vi "Export2Excel.vi"(8 "进度数值":refnum<vi>, 9 "Slide输入":refnum<vi>, 10 "波形数组":cluster{dbl[], dbl[]}[](array[cluster]), 11 "信号名数组":string[](array[string])) -> ()   [LabVIEW 2015]
uses:
  <vilib>/Utility/NIReport.llb/Append Text Table to Report (wrap).vi
  <vilib>/Utility/NIReport.llb/NI_report.lvclass
panel:
  out "进度数值0":string="0%"
  out "水平进度条":u8(slide) scale=0.0..100.0
  # "正在导出至EXCEL，请稍等"
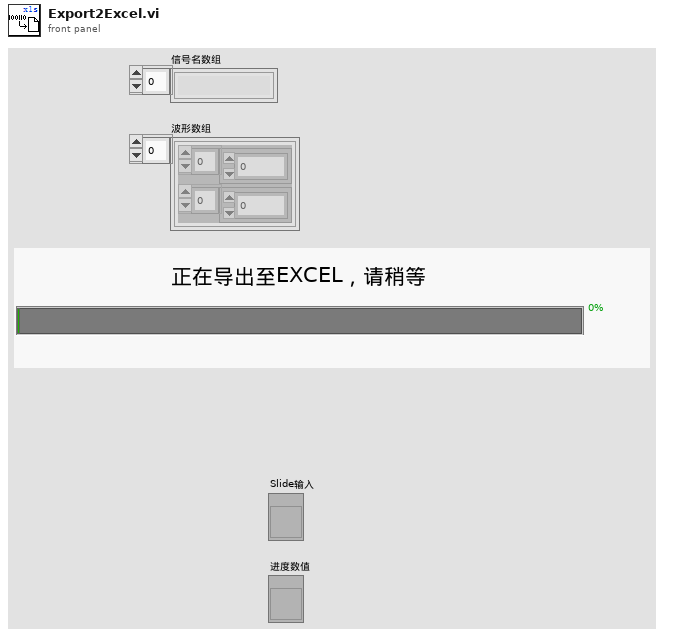
[diagram p1: front panel]
types:
  T1 = enum16{"Standard Report", "HTML", "Word", "Excel"}
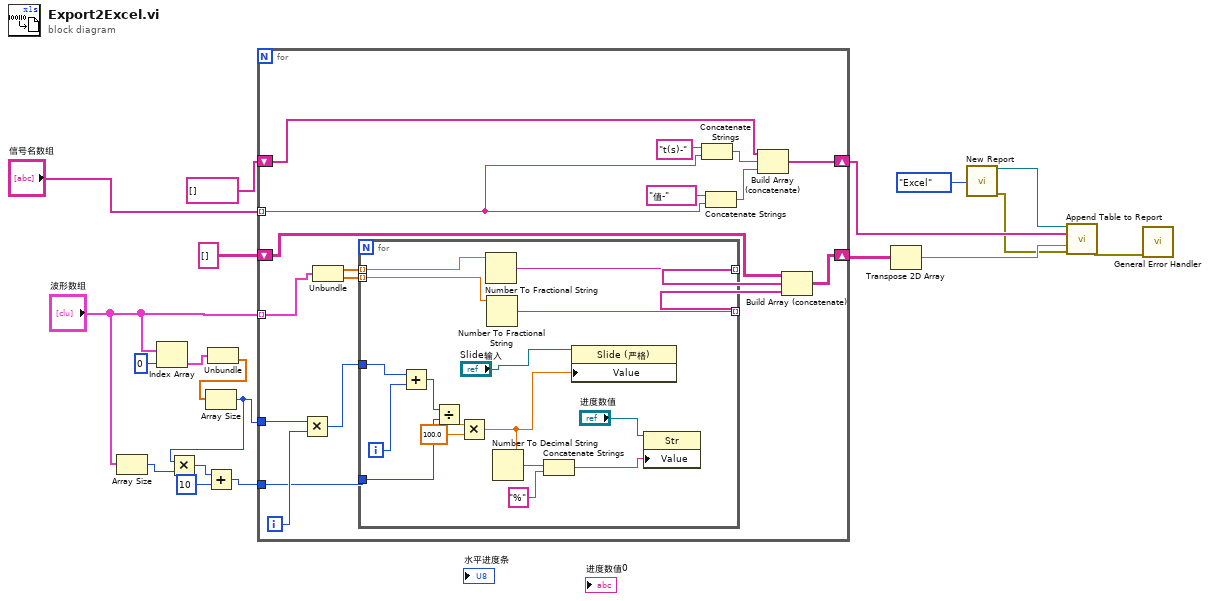
[diagram p0: block diagram]
diagram:
  n1 = Array Size(array="波形数组") -> (size(s)=w7:i32)
  n2 = Index Array(array="波形数组", index=0 ("索引")) -> (element=w9:cluster{dbl[], dbl[]})
  n3 = Unbundle(w9) -> (w8:dbl[])  [unwired: 1 out]
  n4 = Array Size(array=w8) -> (size(s)=w6:i32)
  n5 = Multiply(x=w6, y=w7) -> (x*y=w3:i32)
  n6 = Add(x=w3, y=10) -> (x+y=w2:i32)
  n7 = for {
    tunnel: "波形数组" -> [w33] mode=indexing
    shift-right: [w32] -> w13
    shift-left: string[][] [] -> [w31]
    tunnel: "信号名数组" -> [w27] mode=indexing
    shift-right: [w25] -> w19
    shift-left: string[] [] -> [w24]
    tunnel: w6 -> [w22]
    tunnel: w2 -> [w20]
    i -> [w23]
    n8 = Multiply(x=w22, y=w23) -> (x*y=w21:i32)
    n9 = Unbundle(w33) -> (w37:dbl[], w36:dbl[])
    n10 = for {
      tunnel: w37 -> [w53] mode=indexing
      tunnel: w36 -> [w51] mode=indexing
      tunnel: [w52] -> w35 mode=indexing
      tunnel: [w50] -> w34 mode=indexing
      tunnel: w21 -> [w49]
      tunnel: w20 -> [w46]
      i -> [w48]
      n11 = Add(x=w49, y=w48) -> (x+y=w47:i32)
      n12 = Divide(x=w47, y=w46) -> (x/y=w45:dbl)
      n13 = Multiply(x=w45, y=100.0) -> (x*y=w38:dbl)
      n14 = Number To Fractional String(number=w53) -> (F-format string=w52:string)  [unwired: 3 in]
      n15 = Number To Fractional String(number=w51) -> (F-format string=w50:string)  [unwired: 3 in]
      n16 = Number To Decimal String(number=w38) -> (decimal integer string=w43:string)  [unwired: 1 in]
      n17 = Concatenate Strings(w43, "%" ("字符串")) -> (w40:string)
      n18 = property class="Slide (严格)"(reference="Slide输入", "Value"=w38) -> ()  [unwired: 1 in, 2 out]
      n19 = property class="Str"(reference="进度数值", "Value"=w40) -> ()  [unwired: 1 in, 2 out]
    }
    n20 = Concatenate Strings("t(s)-" ("字符串"), w27) -> (w30:string)
    n21 = Concatenate Strings("值-" ("字符串"), w27) -> (w26:string)
    n22 = Build Array (concatenate)(w24, w30, w26) -> (w25:string[])
    n23 = Build Array (concatenate)(w31, w35, w34) -> (w32:string[][])
  }
  n24 = Transpose 2D Array(2D array=w13) -> (transposed array=w16:string[][])
  n25 = call <vilib>:"New Report.vi"("report type"=T1."Excel") -> ("report out"=w15:refnum<class "NI_report.lvclass">, "error out"=w5:errorcluster)  [unwired: 13 in]
  n26 = call-poly <vilib>:"Append Table to Report.vi"("report in"=w15, "column headers"=w19, "text data"=w16, "error in (no error)"=w5) -> ("error out"=w4:errorcluster)  [unwired: 8 in, 3 out]
  n27 = call <vilib>:"General Error Handler.vi"("error in (no error)"=w4) -> ()  [unwired: 10 in, 5 out]
